vi "Read.vi"(6 "error in":errorcluster, 7 "byte count":u32, 8 "Read command":string="READ?", 9 "VISA resource name":refnum<visa-resource-name>) -> (0 "error out":errorcluster, 2 "Read data":string, 3 "VISA resource name out":refnum<visa-resource-name>)   [LabVIEW 2023, in "Aim TTi 1908P DMM.lvlib"]
uses:
  Aim TTi 1908P DMM.lvlib
  19e38209-455c-425b-9d7c-0b824d84d338.vi
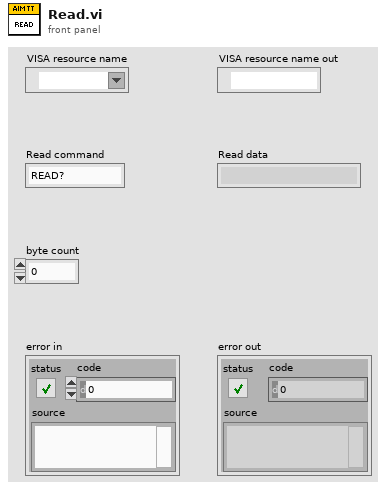
[diagram p1: front panel]
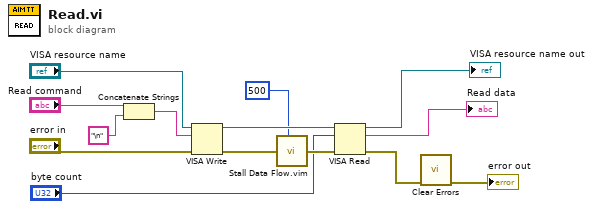
[diagram p0: block diagram]
diagram:
  n1 = Concatenate Strings("Read command", "\n" ("string")) -> (w7:string)
  n2 = VISA Write(VISA resource name="VISA resource name", write buffer=w7, error in (no error)="error in") -> (VISA resource name out=w14:refnum<visa-resource-name>, error out=w13:errorcluster)  [unwired: 1 out]
  n3 = call "Stall Data Flow.vim"("value in"=w13, "milliseconds to wait"=u32 500) -> ("value out"=w12:errorcluster)  [unwired: 1 out]
  n4 = VISA Read(VISA resource name=w14, byte count="byte count", error in (no error)=w12) -> (VISA resource name out=→"VISA resource name out":refnum<visa-resource-name>, read buffer=→"Read data":string, error out=w4:errorcluster)  [unwired: 1 out]
  n5 = call <vilib>:"Clear Errors.vi"("error in (no error)"=w4) -> ("error out"=→"error out":errorcluster)  [unwired: 5 in, 1 out]
